vi "Create DMA Channel.vi"(7 "Original Name":string, 8 "error in (no error)":errorcluster, 9 "Input?":bool, 10 "Name":string, 11 "Section Ref in":T1 format="%.0x") -> (0 "error out":errorcluster, 3 "Parent Ref out":T1 format="%.0x")   [LabVIEW 2019, in "FPGA Addon System Explorer.lvlib"]
uses:
  FPGA Addon System Explorer.lvlib
  <vilib>/NI VeriStand/Custom Device API/Custom Device Item Ref.ctl
  <vilib>/NI VeriStand/Custom Device API/Custom Device Waveform.ctl
  <vilib>/NI VeriStand/Custom Device API/Custom Device Waveform DataType.ctl
  Shared/Constants.vi
  <vilib>/NI VeriStand/Custom Device Tools/Custom Device Utility Library/Custom Device Utility Library.lvlib
  <vilib>/NI VeriStand/Custom Device API/Custom Device API.lvlib
  Shared/FPGA Addon Shared.lvlib
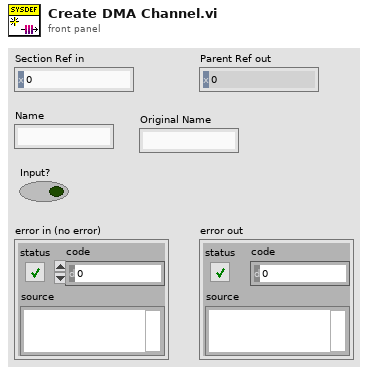
[diagram p1: front panel]
types:
  T1 = typedef "Custom Device API.lvlib/Custom Device Item Ref.ctl" = u64
  T2 = typedef "Custom Device API.lvlib/Custom Device Waveform.ctl" = cluster{"Data Type":T3, "Units":string}
  T3 = typedef "Custom Device API.lvlib/Custom Device Waveform DataType.ctl" = enum16{"Double", "Complex Double"}
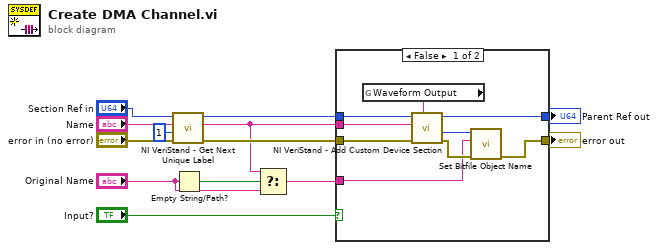
[diagram p0: block diagram]
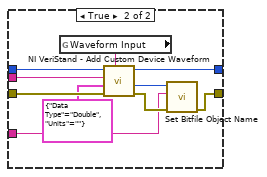
[diagram p2: hidden frame]
diagram:
  n1 = call <vilib>:"NI VeriStand - Get Next Unique Label.vi"("error in (no error)"="error in (no error)", "Start Value (1)"=1, "Label"="Name", "Parent Ref in"="Section Ref in") -> ("error out"=w6:errorcluster, "Label out"=w3:string, "Parent Ref dup"=w7:T1)  [unwired: 4 in, 1 out]
  n2 = Empty String/Path?(string/path="Original Name") -> (empty?=w4:bool)
  n3 = Select(t=w3, s=w4, f="Original Name") -> (s? t:f=w1:string)
  n4 = case shown="False" "Input?" {
    tunnel: [w16 w25] -> w5
    tunnel: w6 -> [w21 w32]
    tunnel: w7 -> [w22 w31]
    tunnel: w3 -> [w18 w27]
    tunnel: [w20 w29] -> w12
    tunnel: w1 -> [w14 w23]
    frame False {
      n5 = global read "Constants.vi" "Waveform Output"() -> (w15:string)
      n6 = call <vilib>:"NI VeriStand - Add Custom Device Section.vi"("GUID (Default Section)"=w15, "error in (no error)"=w21, "Section Name"=w18, "Parent Ref in"=w22) -> ("error out"=w17:errorcluster, "Section Ptr"=w19:T1, "Parent Ref out"=w20:T1)  [unwired: 4 in, 1 out]
      n7 = call "Set Bitfile Object Name.vi"("error in (no error)"=w17, "Name"=w14, "Channel Ref"=w19) -> ("error out"=w16:errorcluster)  [unwired: 8 in]
    }
    frame True {
      n8 = global read "Constants.vi" "Waveform Input"() -> (w24:string)
      n9 = call <vilib>:"NI VeriStand - Add Custom Device Waveform.vi"("GUID (Default Waveform)"=w24, "error in (no error)"=w32, "Waveform"=T2 {"Data Type"=enum."Double", "Units"=""}, "Waveform Name"=w27, "Parent Ref in"=w31) -> ("error out"=w26:errorcluster, "Waveform Ref"=w28:T1, "Parent Ref out"=w29:T1)  [unwired: 3 in, 1 out]
      n10 = call "Set Bitfile Object Name.vi"("error in (no error)"=w26, "Name"=w23, "Channel Ref"=w28) -> ("error out"=w25:errorcluster)  [unwired: 8 in]
    }
  }
  "Parent Ref out" <- w12
  "error out" <- w5
